vi "Sort Scan Parameters.vi"(8 "error in (no error)":errorcluster, 11 "SweepControl":refnum<class "Sweep Control.lvclass">) -> (0 "error out":errorcluster, 1 "Sorted scan parameters":cluster{T5}[](array[cluster])=[{[{"Start"=0.14, "End"=-0.060000000000000005, "Step"=-0.060000000000000005, "Rate"=0.0, "Waveform type"=enum."linear", "wait (ms or K)"=10000.0, "Address"="Dev2/ao0", "channel"=1}]}, {[{"Start"=0.14, "End"=-0.060000000000000005, "Step"=-0.060000000000000005, "Rate"=0.0, "Waveform type"=enum."linear", "wait (ms or K)"=10000.0, "Address"="Dev2/ao0", "channel"=1}]}, {[{"Start"=0.14, "End"=-0.060000000000000005, "Step"=-0.060000000000000005, "Rate"=0.0, "Waveform type"=enum."linear", "wait (ms or K)"=10000.0, "Address"="Dev2/ao0", "channel"=1}, {"Start"=0.14, "End"=-0.060000000000000005, "Step"=-0.060000000000000005, "Rate"=0.0, "Waveform type"=enum."linear", "wait (ms or K)"=10000.0, "Address"="Dev2/ao0", "channel"=1}]}] {"?"."Rate" format="%.2f"; "?"."Step" format="%#_6p"; "?"."End" format="%#_6p"; "?"."Start" format="%#_6p"}, 2 "Sorted scan control":cluster{T7}[](array[cluster])=[{[{"Priority"=enum."Priority 0", "Scan name"=enum."Delay"}]}, {[{"Priority"=enum."Priority 1", "Scan name"=enum."Lockin Amplitude"}]}, {[{"Priority"=enum."Priority 2", "Scan name"=enum."Lockin Bias"}, {"Priority"=enum."Priority 2", "Scan name"=enum."Magnet Field"}]}], 3 "SweepControl":refnum<class "Sweep Control.lvclass">)   [LabVIEW 2019, in "Sweep Control.lvclass"]
uses:
  Sweep Control.lvclass
  Typedefs/ScanControl.ctl
  Typedefs/Cluster - ScanControl.ctl
  Typedefs/Enum - Priority.ctl
  Typedefs/Enum - Action.ctl
  Typedefs/ScanParamters.ctl
  Typedefs/Cluster - ScanParamters.ctl
  Typedefs/Cluster - Sweep Control.ctl
  Typedefs/Enum - PostAction.ctl
  Sweep Control.lvclass/Sweep Control.ctl
panel:
  out "Sorted scan parameters 2":cluster{"Scan parameters 2":T1[]}[](array[cluster]) {"Scan parameters 2"."Rate" format="%.2f"; "Scan parameters 2"."Step" format="%#_6p"; "Scan parameters 2"."End" format="%#_6p"; "Scan parameters 2"."Start" format="%#_6p"}
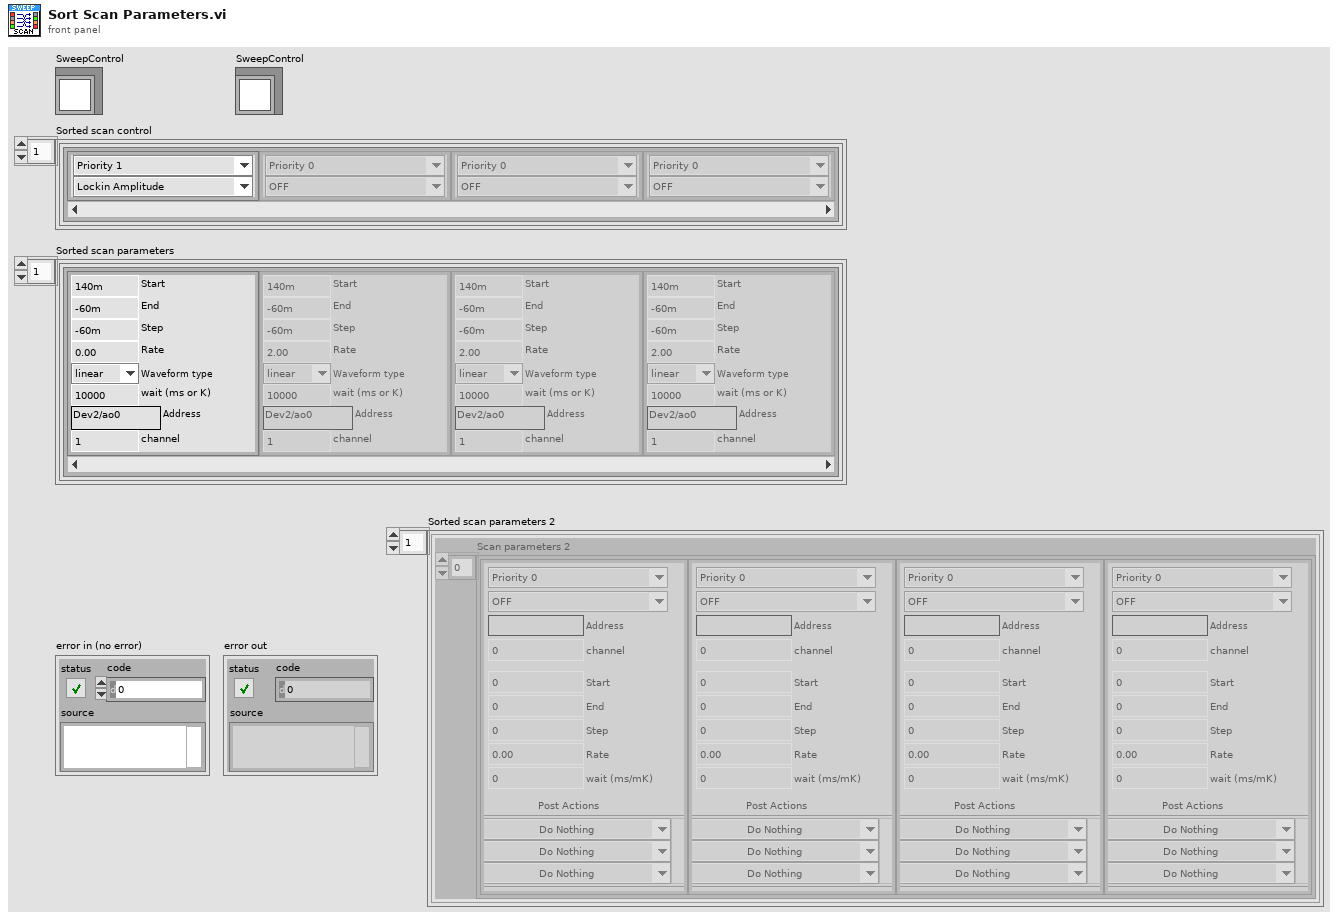
[diagram p1: front panel]
types:
  T1 = typedef "Sweep Control.lvclass/Cluster - Sweep Control.ctl" = cluster{"Start":dbl, "End":dbl, "Step":dbl, "Rate":dbl, "wait (ms/mK)":u32, "Address":string, "Priority":T2, "Scan name":T3, "Post Actions":T4[], "channel":i32}
  T2 = typedef "Sweep Control.lvclass/Enum - Priority.ctl" = enum16{"Priority 0", "Priority 1", "Priority 2", "Priority 3", "Priority 4", "Priority 5"}
  T3 = typedef "Sweep Control.lvclass/Enum - Action.ctl" = enum16{"OFF", "time", "Lockin Amplitude", "Lockin Frequency", "Lockin Bias", "Delay", "Strain", "DAQ Bias", "Magnet Field", "Temperature", "MW f1", "MW f2", "MW Amplitude1", "MW Amplitude2"}
  T4 = typedef "Sweep Control.lvclass/Enum - PostAction.ctl" = enum16{"Do Nothing", "Wait (time)", "Wait (Temperature)", "Wait (<T ; B sweep)", "Wait (Magnet)"}
  T5 = typedef "Sweep Control.lvclass/ScanParamters.ctl" = T6[]
  T6 = typedef "Sweep Control.lvclass/Cluster - ScanParamters.ctl" = cluster{"Start":dbl, "End":dbl, "Step":dbl, "Rate":dbl, "Waveform type":enum16{"linear", "triangle", "power"}, "wait (ms or K)":dbl, "Address":string, "channel":i32}
  T7 = typedef "Sweep Control.lvclass/ScanControl.ctl" = T8[]
  T8 = typedef "Sweep Control.lvclass/Cluster - ScanControl.ctl" = cluster{"Priority":T2, "Scan name":T3}
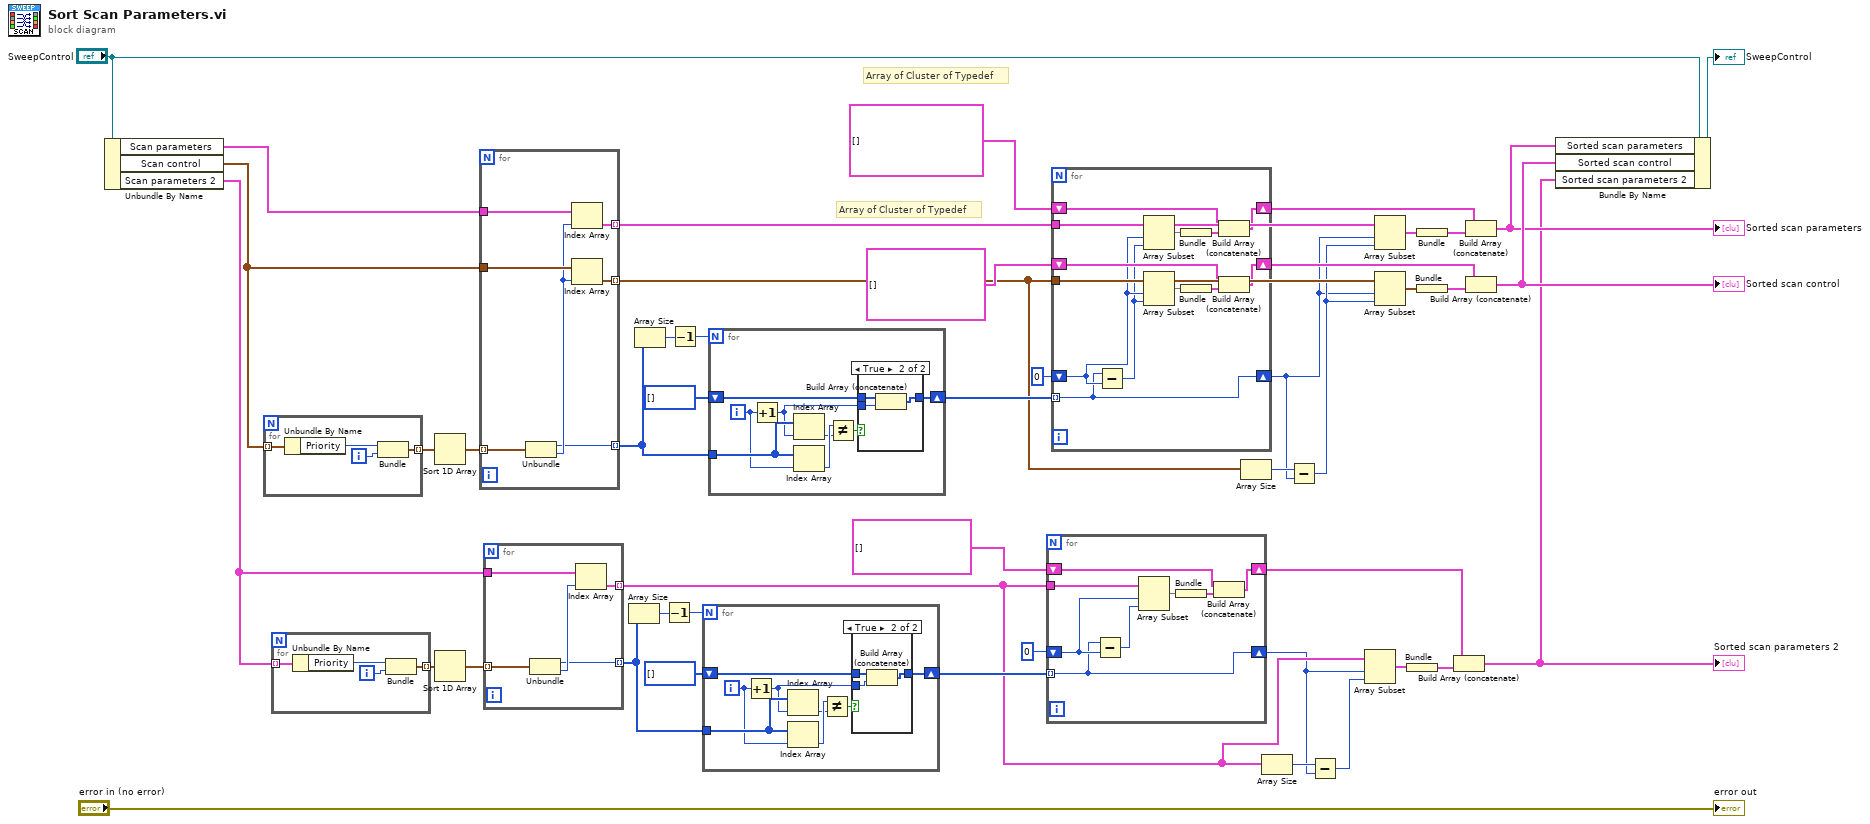
[diagram p0: block diagram]
diagram:
  # "Array of Cluster of Typedef"
  # "Array of Cluster of Typedef"
  n1 = Unbundle By Name("SweepControl") -> ("Scan parameters"=w1:T5, "Scan control"=w3:T7, "Scan parameters 2"=w2:T1[])
  n2 = for {
    tunnel: w3 -> [w47] mode=indexing
    tunnel: [w50] -> w46 mode=indexing
    i -> [w48]
    n3 = Unbundle By Name(w47) -> ("Priority"=w49:T2)
    n4 = Bundle("Priority"=w49, w48) -> (w50:cluster{"Priority":T2, i32})  [unwired: 1 in]
  }
  n5 = for {
    tunnel: w2 -> [w51] mode=indexing
    tunnel: [w54] -> w21 mode=indexing
    i -> [w52]
    n6 = Unbundle By Name(w51) -> ("Priority"=w53:T2)
    n7 = Bundle("Priority"=w53, w52) -> (w54:cluster{"Priority":T2, i32})  [unwired: 1 in]
  }
  n8 = Sort 1D Array(array=w46) -> (sorted array=w45:cluster{"Priority":T2, i32}[])
  n9 = Sort 1D Array(array=w21) -> (sorted array=w20:cluster{"Priority":T2, i32}[])
  n10 = for {
    tunnel: w45 -> [w61] mode=indexing
    tunnel: w3 -> [w60]
    tunnel: [w59] -> w36 mode=indexing
    tunnel: w1 -> [w58]
    tunnel: [w57] -> w32 mode=indexing
    tunnel: [w55] -> w4 mode=indexing
    n11 = Unbundle(w61) -> ("Priority"=w55:T2, w56:i32)
    n12 = Index Array(array=w58, index=w56) -> (element=w57:T6)
    n13 = Index Array(array=w60, index=w56) -> (element=w59:T8)
  }
  n14 = for {
    tunnel: w20 -> [w66] mode=indexing
    tunnel: w2 -> [w65]
    tunnel: [w64] -> w12 mode=indexing
    tunnel: [w62] -> w5 mode=indexing
    n15 = Unbundle(w66) -> ("Priority"=w62:T2, w63:i32)
    n16 = Index Array(array=w65, index=w63) -> (element=w64:T1)
  }
  n17 = Array Size(array=w5) -> (size(s)=w17:i32)
  n18 = Array Size(array=w4) -> (size(s)=w44:i32)
  n19 = Decrement(x=w17) -> (x-1=w18:i32)
  n20 = Decrement(x=w44) -> (x-1=w43:i32)
  n21 = for {
    N: w18 -> [_]
    tunnel: w5 -> [w74]
    shift-right: [w70] -> w15
    shift-left: i32[] [] -> [w69]
    i -> [w67]
    n22 = Increment(x=w67) -> (x+1=w68:i32)
    n23 = Index Array(array=w74, index=w68) -> (element=w71:T2)
    n24 = Index Array(array=w74, index=w67) -> (element=w73:T2)
    n25 = Not Equal?(x=w73, y=w71) -> (x != y?=w72:bool)
    n26 = case shown="True" w72 {
      tunnel: [w75 w78] -> w70
      tunnel: w69 -> [w75 w77]
      tunnel: w68 -> [_ w76]
      frame False {
      }
      frame True {
        n27 = Build Array (concatenate)(w77, w76) -> (w78:i32[])
      }
    }
  }
  n28 = for {
    N: w43 -> [_]
    tunnel: w4 -> [w86]
    shift-right: [w82] -> w40
    shift-left: i32[] [] -> [w81]
    i -> [w79]
    n29 = Increment(x=w79) -> (x+1=w80:i32)
    n30 = Index Array(array=w86, index=w80) -> (element=w83:T2)
    n31 = Index Array(array=w86, index=w79) -> (element=w85:T2)
    n32 = Not Equal?(x=w85, y=w83) -> (x != y?=w84:bool)
    n33 = case shown="True" w84 {
      tunnel: [w87 w88] -> w82
      tunnel: w81 -> [w87 w90]
      tunnel: w80 -> [_ w89]
      frame False {
      }
      frame True {
        n34 = Build Array (concatenate)(w90, w89) -> (w88:i32[])
      }
    }
  }
  n35 = for {
    tunnel: w15 -> [w91] mode=indexing
    shift-right: [w91] -> w8
    shift-left: 0 -> [w92]
    tunnel: w12 -> [w98]
    shift-right: [w95] -> w9
    shift-left: cluster{"Scan parameters 2":T1[]}[] [] -> [w94]
    n36 = Subtract(x=w91, y=w92) -> (x-y=w97:i32)
    n37 = Array Subset(array=w98, index=w92, length=w97) -> (w96:T1[])
    n38 = Bundle(w96) -> (w93:cluster{T1[]})  [unwired: 1 in]
    n39 = Build Array (concatenate)(w94, w93) -> (w95:cluster{"Scan parameters 2":T1[]}[])
  }
  n40 = for {
    tunnel: w40 -> [w99] mode=indexing
    shift-right: [w111] -> w39
    shift-left: cluster{"Scan control":T7}[] [] -> [w110]
    tunnel: w36 -> [w109]
    shift-right: [w99] -> w30
    shift-left: 0 -> [w105]
    tunnel: w32 -> [w106]
    shift-right: [w102] -> w27
    shift-left: cluster{"Scan parameters":T5}[] [] -> [w101]
    n41 = Subtract(x=w99, y=w105) -> (x-y=w104:i32)
    n42 = Array Subset(array=w106, index=w105, length=w104) -> (w103:T6[])
    n43 = Array Subset(array=w109, index=w105, length=w104) -> (w108:T8[])
    n44 = Bundle(w103) -> (w100:cluster{T6[]})  [unwired: 1 in]
    n45 = Bundle(w108) -> (w107:cluster{T8[]})  [unwired: 1 in]
    n46 = Build Array (concatenate)(w101, w100) -> (w102:cluster{"Scan parameters":T5}[])
    n47 = Build Array (concatenate)(w110, w107) -> (w111:cluster{"Scan control":T7}[])
  }
  n48 = Array Size(array=w36) -> (size(s)=w37:i32)
  n49 = Array Size(array=w12) -> (size(s)=w13:i32)
  n50 = Subtract(x=w37, y=w30) -> (x-y=w31:i32)
  n51 = Subtract(x=w13, y=w8) -> (x-y=w7:i32)
  n52 = Array Subset(array=w12, index=w8, length=w7) -> (w11:T1[])
  n53 = Array Subset(array=w32, index=w30, length=w31) -> (w33:T6[])
  n54 = Array Subset(array=w36, index=w30, length=w31) -> (w35:T8[])
  n55 = Bundle(w11) -> (w10:cluster{T1[]})  [unwired: 1 in]
  n56 = Bundle(w33) -> (w29:cluster{T6[]})  [unwired: 1 in]
  n57 = Bundle(w35) -> (w34:cluster{T8[]})  [unwired: 1 in]
  n58 = Build Array (concatenate)(w9, w10) -> (w6:cluster{"Scan parameters 2":T1[]}[])
  "Sorted scan parameters 2" <- w6
  n59 = Build Array (concatenate)(w27, w29) -> (w24:cluster{"Scan parameters":T5}[])
  "Sorted scan parameters" <- w24
  n60 = Build Array (concatenate)(w39, w34) -> (w25:cluster{"Scan control":T7}[])
  "Sorted scan control" <- w25
  n61 = Bundle By Name(cluster="SweepControl", "Sorted scan parameters"=w24, "Sorted scan control"=w25, "Sorted scan parameters 2"=w6) -> (→"SweepControl":refnum<class "Sweep Control.lvclass">)
  "error out" <- "error in (no error)"
